vi "Virtual Oscilloscope.vi"() -> ()   [LabVIEW 2017]
uses:
  Control 3.ctl
  Virt.Scope.ctl
  <instrlib>/Tektronix TDS 200 1000 2000 Series/Public/Configure/Configure Trigger (Edge).vi
  <instrlib>/Tektronix TDS 200 1000 2000 Series/Tektronix TDS 200 1000 2000 Series.lvlib
panel:
  in  "Rising/Falling":u16(ring) items=["Rising", "Falling"]
  out "Waveform Graph 2":waveform(dbl)(graph)={"t0"=timestamp(-0.050000000000000044 s since 1904-01-01), "dt"=4e-05, "Y"=[]}
  out "Waveform Graph":waveform(dbl)(graph)
  in  "Meas. Type":T1
  out "Measurement":dbl=21.349275589
  in  "stop":bool
  in  "Measure":bool
  in  "Voltage Scale 2":dbl(ring)=5.0 items=["50 V"=50.0, "20 V"=20.0, "10 V"=10.0, "5 V"=5.0, "2 V"=2.0, "1 V"=1.0, "500 mV"=0.5, "200 mV"=0.2, "100 mV"=0.1, "50 mV"=0.05, "20 mV"=0.02]
  in  "Voltage Scale 1":dbl(ring)=10.0 items=["50 V"=50.0, "20 V"=20.0, "10 V"=10.0, "5 V"=5.0, "2 V"=2.0, "1 V"=1.0, "500 mV"=0.5, "200 mV"=0.2, "100 mV"=0.1, "50 mV"=0.05, "20 mV"=0.02]
  in  "Horz Trigger":dbl min=-1.0 max=1.0 step=0.001
  in  "Vert Trigger":dbl min=-200.0 max=200.0 step=1.0
  in  "Time Scale":dbl(ring)=0.01 items=["50 s"=50.0, "25 s"=25.0, "10 s"=10.0, "5 s"=5.0, "2.50 s"=2.5, "1 s"=1.0, "500 ms"=0.5, "250 ms"=0.25, "100 ms"=0.1, "50 ms"=0.05, "25 ms"=0.025, "10 ms"=0.01, "5 ms"=0.005, "2.50 ms"=0.0025, "1 ms"=0.001, "500 us"=0.0005, "250 us"=0.00025, "100 us"=0.0001, "50 us"=5e-05, "25 us"=2.5e-05, "10 us"=1e-05, "5 us"=5e-06, "2.50 us"=2.5e-06, "1 us"=1e-06, "500 ns"=5e-07, "250 ns"=2.5e-07, "100 ns"=1e-07, "50 ns"=5e-08, "25 ns"=2.5e-08, "10 ns"=1e-08, "5 ns"=5e-09]
  in  "Auto Set":bool
  # "Vertical"
  # "Horizontal"
  # "Ch 1"
  # "Ch 2"
  # "s"
  # "V"
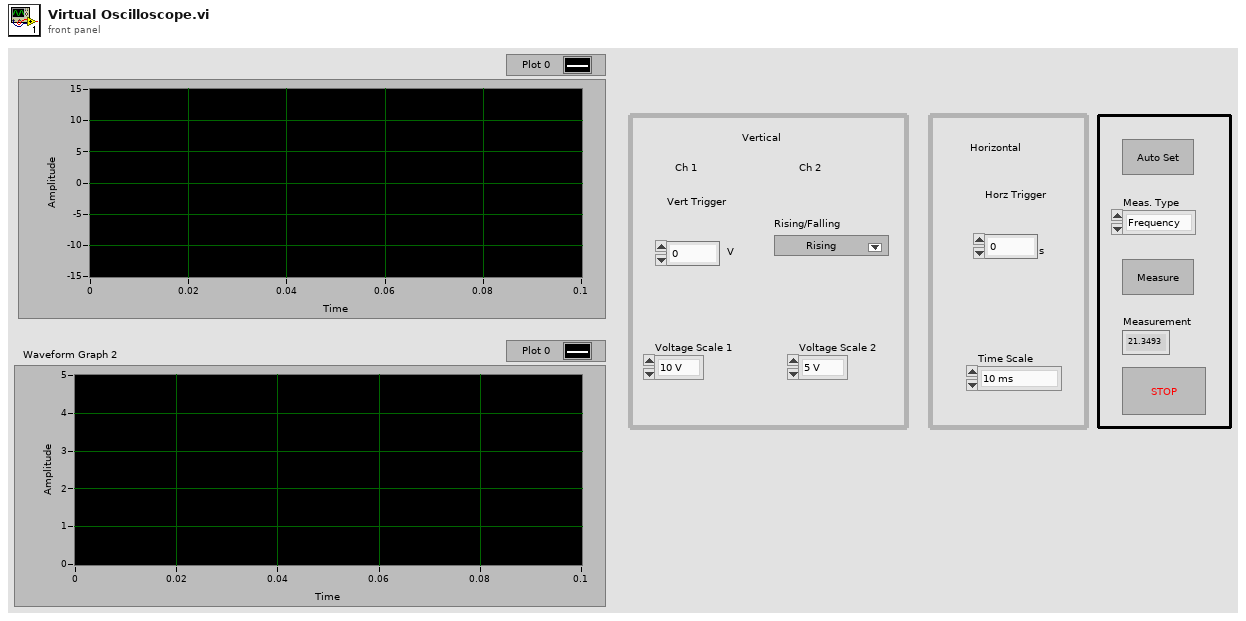
[diagram p1: front panel]
types:
  T1 = typedef "Control 3.ctl" = enum16{"Frequency", "Period", "PK-PK", "Cycle RMS"}
  T2 = typedef "Virt.Scope.ctl" = enum16{"Initialize", "Wait For UI", "Update", "Auto Set", "Read", "Display", "Stop"}
  T3 = cluster{"Baud Rate":u32, "Parity":u16, "Stop Bits":u16, "Flow Control":u16}
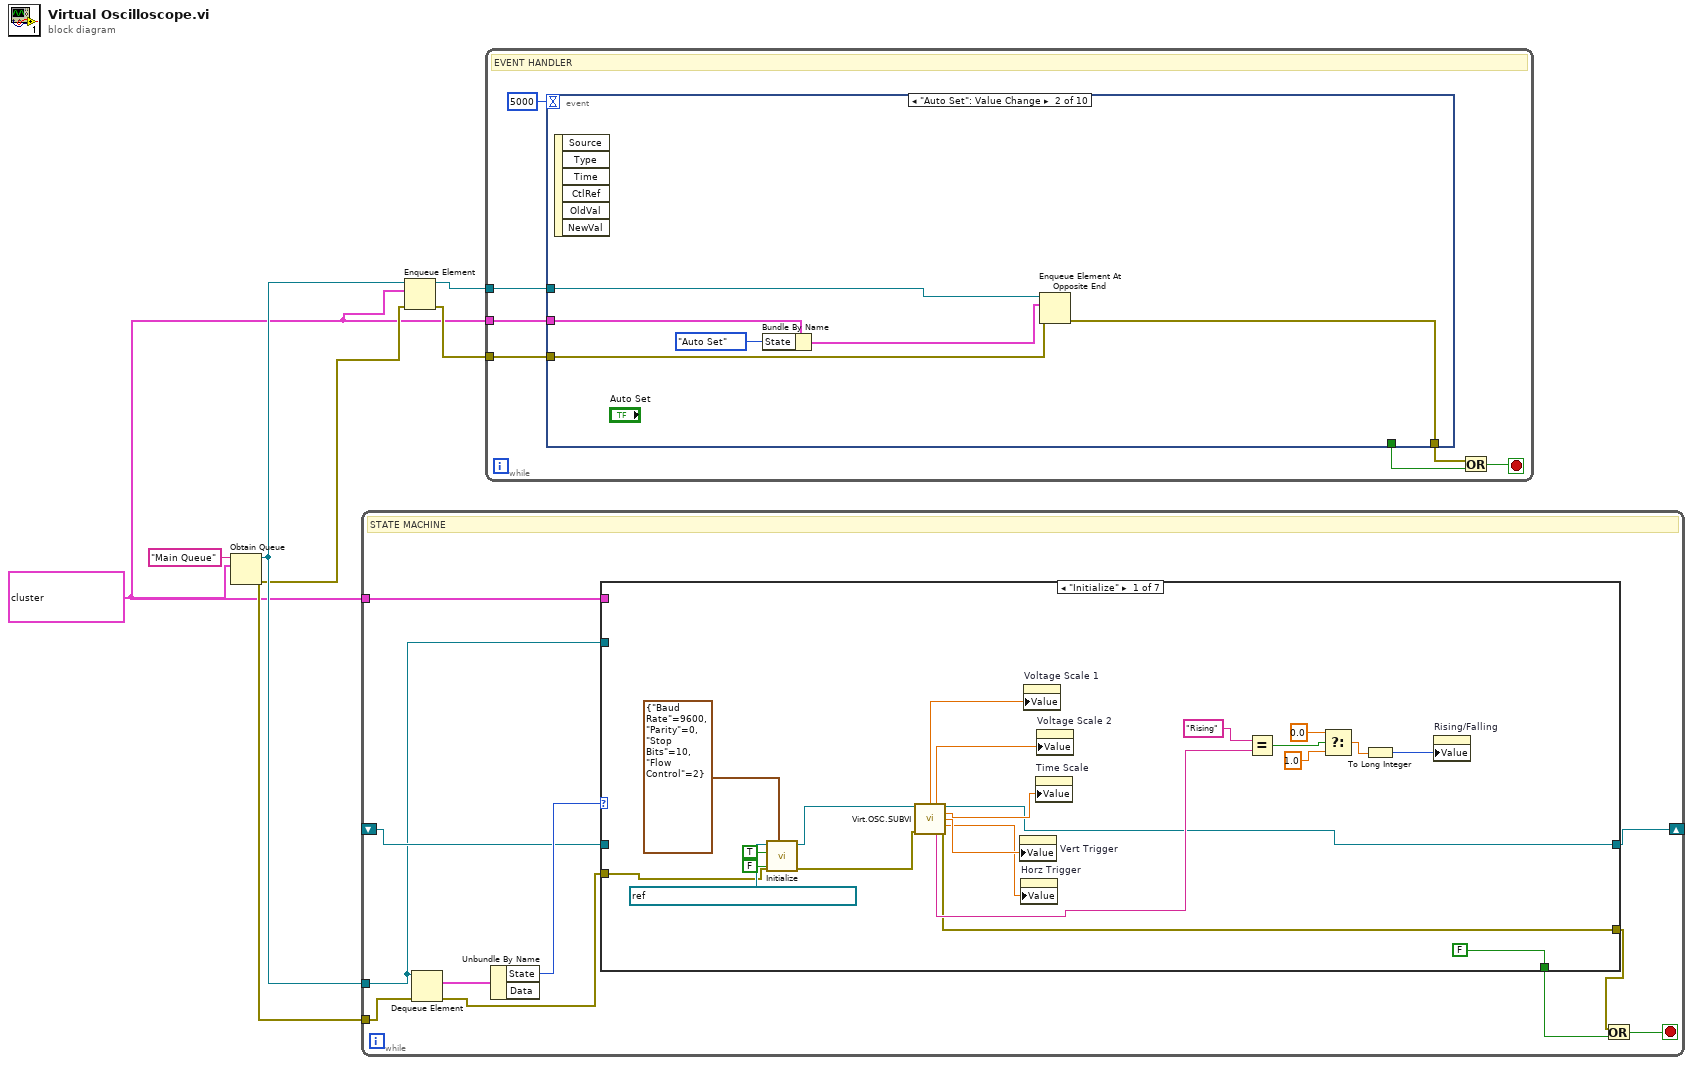
[diagram p0: block diagram]
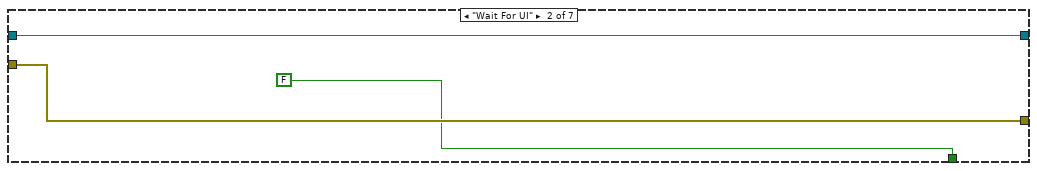
[diagram p2: hidden frame]
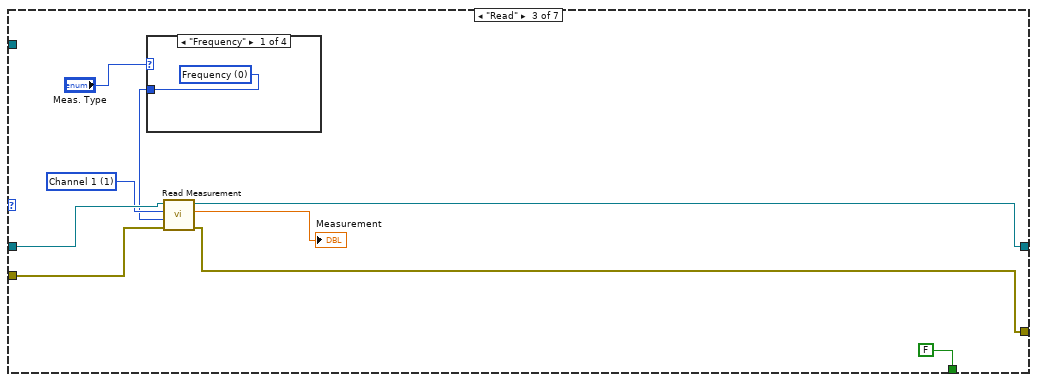
[diagram p3: hidden frame]
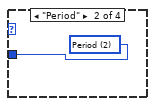
[diagram p4: hidden frame]
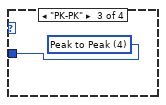
[diagram p5: hidden frame]
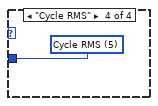
[diagram p6: hidden frame]
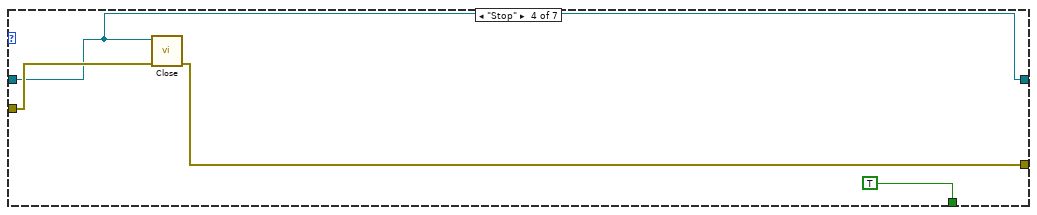
[diagram p7: hidden frame]
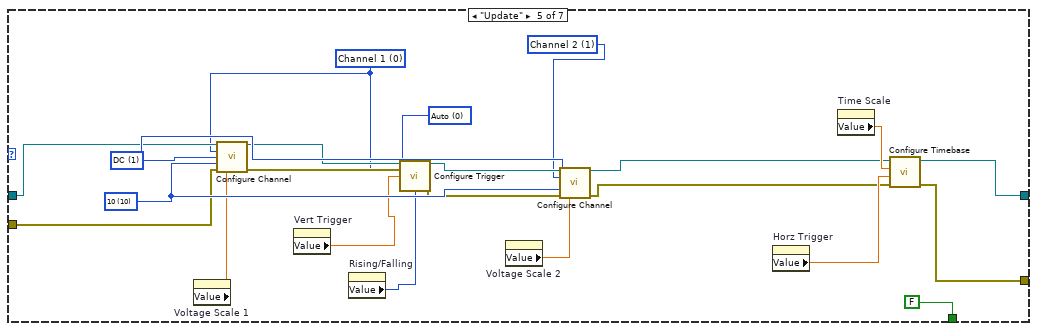
[diagram p8: hidden frame]
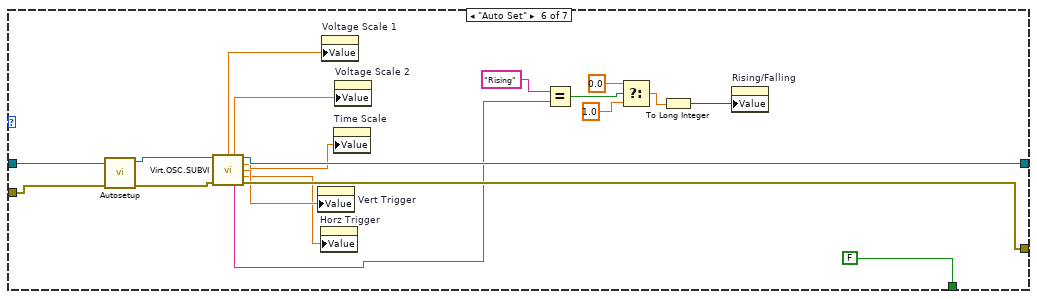
[diagram p9: hidden frame]
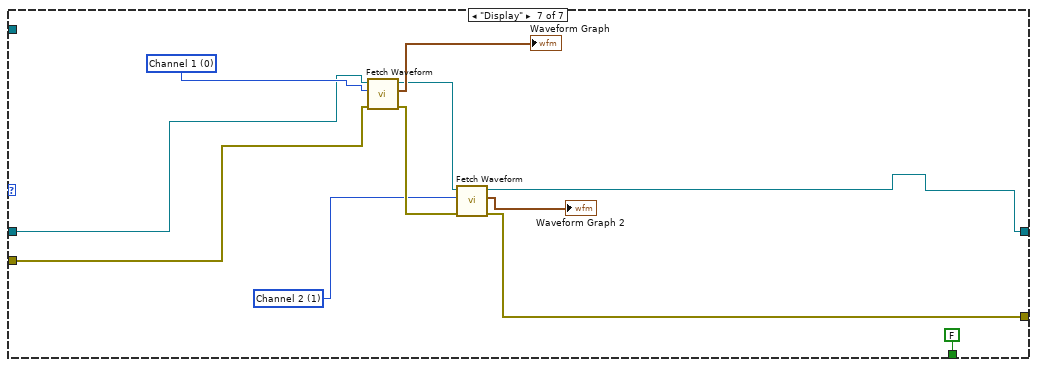
[diagram p10: hidden frame]
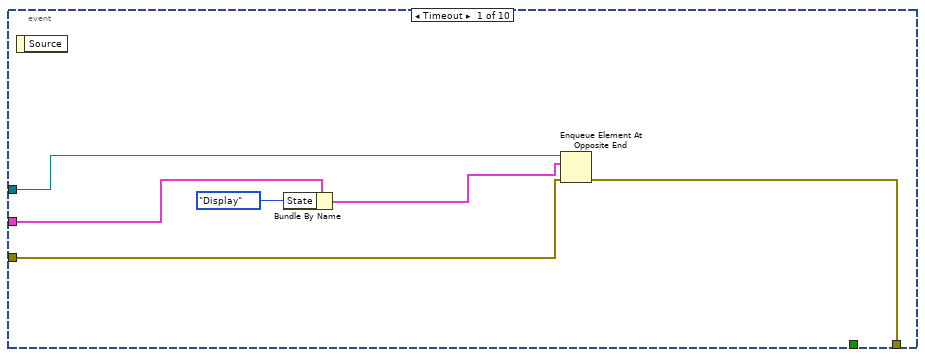
[diagram p11: hidden frame]
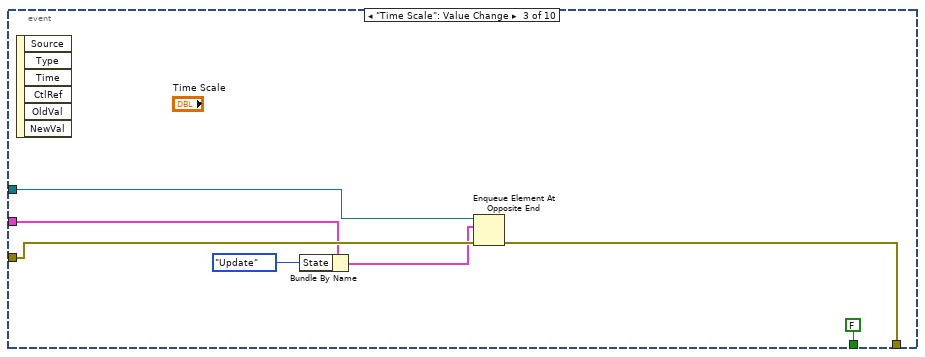
[diagram p12: hidden frame]
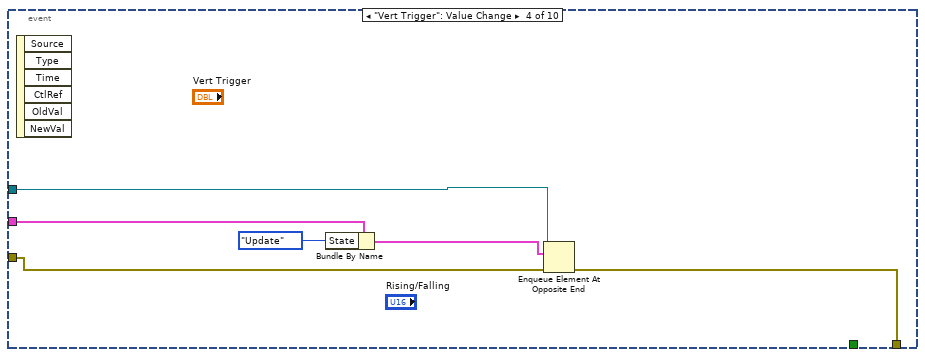
[diagram p13: hidden frame]
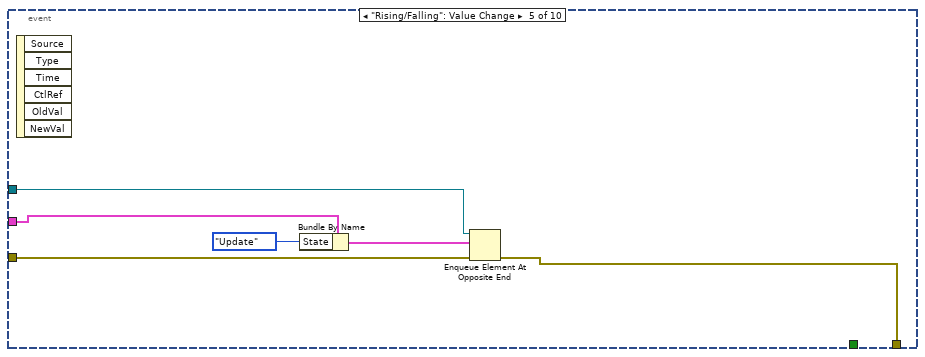
[diagram p14: hidden frame]
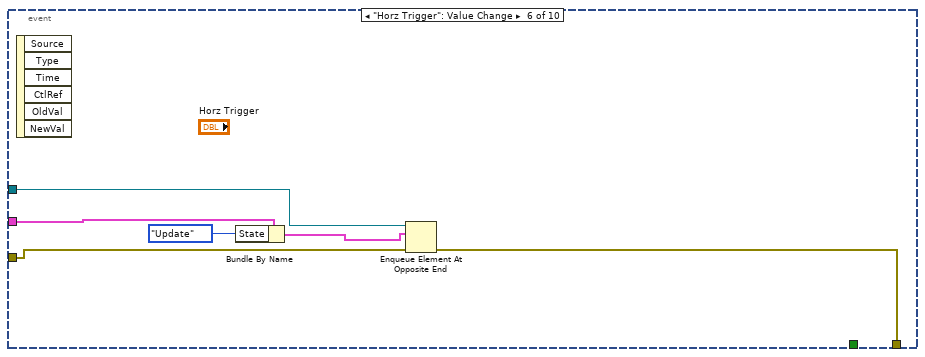
[diagram p15: hidden frame]
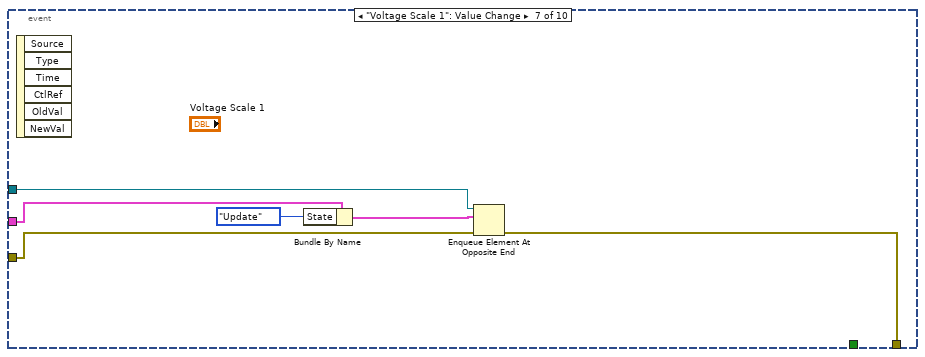
[diagram p16: hidden frame]
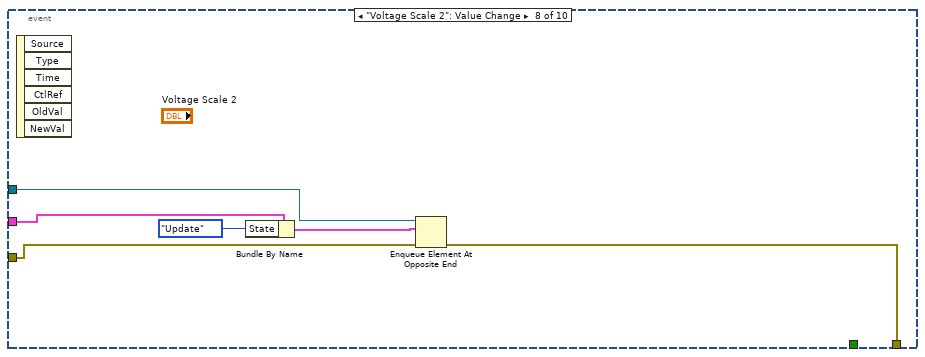
[diagram p17: hidden frame]
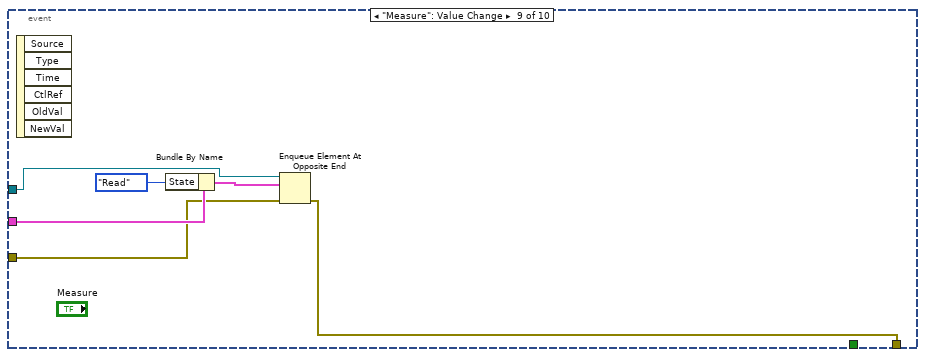
[diagram p18: hidden frame]
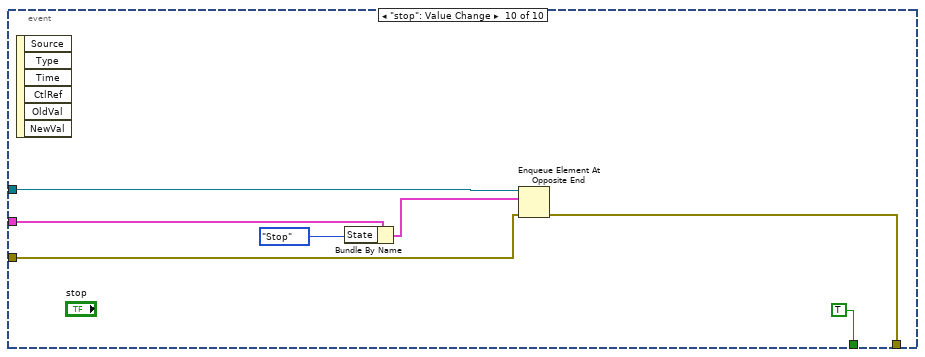
[diagram p19: hidden frame]
diagram:
  w1 = cluster{"Data":variant, "State":T2} {"Data"=variant, "State"=enum."Initialize"}
  n1 = Obtain Queue(name (unnamed)="Main Queue", element data type=w1) -> (queue out=w5:refnum<queue>, error out=w3:errorcluster)  [unwired: 3 in, 1 out]
  n2 = while {
    tunnel: w3 -> [w16]
    tunnel: w5 -> [w9]
    shift-right: [w7] -> _
    shift-left: _ -> [w11]
    tunnel: w1 -> [w8]
    stop <- w17 stop-if-true
    # "STATE MACHINE"
    n3 = Dequeue Element(queue=w9, error in (no error)=w16) -> (element=w15:cluster{"Data":variant, "State":T2}, error out=w13:errorcluster)  [unwired: 1 in, 2 out]
    n4 = Unbundle By Name(w15) -> ("State"=w14:T2)  [unwired: 1 out]
    n5 = case shown="\"Initialize\"" w14 {
      tunnel: w13 -> [w36 w41 w46 w59 w72 w98 w108]
      tunnel: [w19 w41 w44 w58 w71 w94 w102] -> w12
      tunnel: [w20 w42 w45 w56 w78 w95 w103] -> w7
      tunnel: w11 -> [_ w42 w51 w56 w73 w99 w109]
      tunnel: [FALSE FALSE FALSE TRUE FALSE FALSE FALSE] -> w10
      tunnel: w9 -> [_ _ _ _ _ _ _]
      tunnel: w8 -> [_ _ _ _ _ _ _]
      frame "Initialize" {
        n6 = call <instrlib>:"Initialize.vi"("Serial Configuration"=T3 {"Baud Rate"=9600, "Parity"=0, "Stop Bits"=10, "Flow Control"=2}, "error in (no error)"=w36, "Reset? (T: Yes)"=FALSE, "ID Query? (T: Yes)"=TRUE, "VISA resource name"=refnum<visa-resource-name> "USB0::0x0699::0x03A0::C014023::INSTR") -> ("error out"=w21:errorcluster, "VISA resource name out"=w22:refnum<visa-resource-name>)  [unwired: 5 in]
        n7 = call "Virt.OSC.SUBVI.vi"("VISA resource name"=w22, "Error In"=w21) -> ("Channel 1 Scale"=w33:dbl, "Channel 2 Scale"=w32:dbl, "VISA resource name out"=w20:refnum<visa-resource-name>, "Time Base"=w31:dbl, "vertical trigger"=w30:dbl, "horziontal trigger"=w18:dbl, "rise/fall"=w29:string, "Error Out"=w19:errorcluster)  [unwired: 6 in]
        n8 = property on="Vert Trigger" class="DigNum (strict)"("Value"=w30) -> ()  [unwired: 2 in, 2 out]
        n9 = property on="Horz Trigger" class="DigNum (strict)"("Value"=w18) -> ()  [unwired: 2 in, 2 out]
        n10 = property on="Voltage Scale 1" class="Ring (strict)"("Value"=w33) -> ()  [unwired: 2 in, 2 out]
        n11 = property on="Time Scale" class="Ring (strict)"("Value"=w31) -> ()  [unwired: 2 in, 2 out]
        n12 = property on="Voltage Scale 2" class="Ring (strict)"("Value"=w32) -> ()  [unwired: 2 in, 2 out]
        n13 = Equal?(x="Rising", y=w29) -> (x = y?=w28:bool)
        n14 = Select(t=0.0, s=w28, f=1.0) -> (s? t:f=w27:dbl)
        n15 = To Long Integer(number=w27) -> (32bit integer=w26:i32)
        n16 = property on="Rising/Falling" class="Ring (strict)"("Value"=w26) -> ()  [unwired: 2 in, 2 out]
      }
      frame "Wait For UI" {
      }
      frame "Read" {
        w50 = 1 items=["Channel 1"=1, "Channel 2"=2, "Channel 3"=3, "Channel 4"=4] ("Channel (1: Channel 1)")
        n17 = case shown="\"Frequency\"" "Meas. Type" {
          tunnel: [w52 w53 w54 w55] -> w47
          frame "Frequency" {
            w52 = 0 items=["Frequency", "Mean", "Period", "Pulse Duty", "Peak to Peak", "Cycle RMS", "Minimum", "Maximum", "Rise Time", "Fall Time", "Positive Width", "Negative Width", "Amplitude", "Cycle Mean", "High", "Low", "Negative Duty", "Positive Overshoot", "Negative Overshoot", "Cursor Mean", "Burst Width", "Positive Pulse Count", "Negative Pulse Count", "Rising Edge Count", "Falling Edge Count", "Area", "Cycle Area", "RMS", "Cursor RMS"] ("Measurement Type (0: Frequency)")
          }
          frame "Period" {
            w53 = 2 items=["Frequency", "Mean", "Period", "Pulse Duty", "Peak to Peak", "Cycle RMS", "Minimum", "Maximum", "Rise Time", "Fall Time", "Positive Width", "Negative Width", "Amplitude", "Cycle Mean", "High", "Low", "Negative Duty", "Positive Overshoot", "Negative Overshoot", "Cursor Mean", "Burst Width", "Positive Pulse Count", "Negative Pulse Count", "Rising Edge Count", "Falling Edge Count", "Area", "Cycle Area", "RMS", "Cursor RMS"] ("Measurement Type (0: Frequency)")
          }
          frame "PK-PK" {
            w54 = 4 items=["Frequency", "Mean", "Period", "Pulse Duty", "Peak to Peak", "Cycle RMS", "Minimum", "Maximum", "Rise Time", "Fall Time", "Positive Width", "Negative Width", "Amplitude", "Cycle Mean", "High", "Low", "Negative Duty", "Positive Overshoot", "Negative Overshoot", "Cursor Mean", "Burst Width", "Positive Pulse Count", "Negative Pulse Count", "Rising Edge Count", "Falling Edge Count", "Area", "Cycle Area", "RMS", "Cursor RMS"] ("Measurement Type (0: Frequency)")
          }
          frame "Cycle RMS" {
            w55 = 5 items=["Frequency", "Mean", "Period", "Pulse Duty", "Peak to Peak", "Cycle RMS", "Minimum", "Maximum", "Rise Time", "Fall Time", "Positive Width", "Negative Width", "Amplitude", "Cycle Mean", "High", "Low", "Negative Duty", "Positive Overshoot", "Negative Overshoot", "Cursor Mean", "Burst Width", "Positive Pulse Count", "Negative Pulse Count", "Rising Edge Count", "Falling Edge Count", "Area", "Cycle Area", "RMS", "Cursor RMS"] ("Measurement Type (0: Frequency)")
          }
        }
        n18 = call <instrlib>:"Read Measurement.vi"("error in (no error)"=w46, "Measurement Type (0: Frequency)"=w47, "Channel (1: Channel 1)"=w50, "VISA resource name"=w51) -> ("error out"=w44:errorcluster, "Measurement"=→"Measurement":dbl, "VISA resource name out"=w45:refnum<visa-resource-name>)  [unwired: 4 in, 1 out]
      }
      frame "Stop" {
        n19 = call <instrlib>:"Close.vi"("error in (no error)"=w59, "VISA resource name"=w56) -> ("error out"=w58:errorcluster)  [unwired: 9 in]
      }
      frame "Update" {
        w63 = 0 items=["Auto", "Normal"] ("Trigger Mode (0: Auto)")
        w64 = 1 items=["Channel 1", "Channel 2", "Channel 3", "Channel 4", "Math", "Reference A", "Reference B", "Reference C", "Reference D"] ("Channel (0: Channel 1)")
        w79 = 10 items=["1"=1, "10"=10, "20"=20, "50"=50, "100"=100, "500"=500, "1000"=1000] ("Probe Attenuation (10: 10X)")
        w80 = 1 items=["AC", "DC", "Ground"] ("Vertical Coupling (1: DC)")
        w66 = 0 items=["Channel 1", "Channel 2", "Channel 3", "Channel 4", "Math", "Reference A", "Reference B", "Reference C", "Reference D"] ("Channel (0: Channel 1)")
        n20 = property on="Voltage Scale 1" class="Ring (strict)"() -> ("Value"=w77:dbl)  [unwired: 2 in, 2 out]
        n21 = call <instrlib>:"Configure Channel.vi"("VISA resource name"=w73, "Channel (0: Channel 1)"=w66, "Vertical Coupling (1: DC)"=w80, "Probe Attenuation (10: 10X)"=w79, "error in (no error)"=w72, "Vertical Range (10.0 V/div)"=w77) -> ("VISA resource name out"=w70:refnum<visa-resource-name>, "error out"=w69:errorcluster)  [unwired: 8 in]
        n22 = property on="Vert Trigger" class="DigNum (strict)"() -> ("Value"=w65:dbl)  [unwired: 2 in, 2 out]
        n23 = property on="Rising/Falling" class="Ring (strict)"() -> ("Value"=w62:u16)  [unwired: 2 in, 2 out]
        n24 = call-poly <instrlib>:"Configure Trigger.vi"("VISA resource name"=w70, "Trigger Source (0: Channel 1)"=w66, "Trigger Level (0.0 V)"=w65, "Trigger Mode (0: Auto)"=w63, "error in (no error)"=w69, "Trigger Slope (0: Rising)"=w62) -> ("VISA resource name out"=w67:refnum<visa-resource-name>, "error out"=w68:errorcluster)  [unwired: 8 in]
        n25 = property on="Voltage Scale 2" class="Ring (strict)"() -> ("Value"=w76:dbl)  [unwired: 2 in, 2 out]
        n26 = call <instrlib>:"Configure Channel.vi"("VISA resource name"=w67, "Channel (0: Channel 1)"=w64, "Vertical Coupling (1: DC)"=w80, "Probe Attenuation (10: 10X)"=w79, "error in (no error)"=w68, "Vertical Range (10.0 V/div)"=w76) -> ("VISA resource name out"=w61:refnum<visa-resource-name>, "error out"=w60:errorcluster)  [unwired: 8 in]
        n27 = property on="Horz Trigger" class="DigNum (strict)"() -> ("Value"=w75:dbl)  [unwired: 2 in, 2 out]
        n28 = property on="Time Scale" class="Ring (strict)"() -> ("Value"=w74:dbl)  [unwired: 2 in, 2 out]
        n29 = call <instrlib>:"Configure Timebase.vi"("error in (no error)"=w60, "Position (0.0 s)"=w75, "Timebase (0.0005 s)"=w74, "VISA resource name"=w61) -> ("error out"=w71:errorcluster, "VISA resource name out"=w78:refnum<visa-resource-name>)  [unwired: 6 in]
      }
      frame "Auto Set" {
        n30 = call <instrlib>:"Autosetup.vi"("error in (no error)"=w98, "VISA resource name"=w99) -> ("error out"=w96:errorcluster, "VISA resource name out"=w97:refnum<visa-resource-name>)  [unwired: 8 in]
        n31 = call "Virt.OSC.SUBVI.vi"("VISA resource name"=w97, "Error In"=w96) -> ("Channel 1 Scale"=w93:dbl, "Channel 2 Scale"=w92:dbl, "VISA resource name out"=w95:refnum<visa-resource-name>, "Time Base"=w91:dbl, "vertical trigger"=w90:dbl, "horziontal trigger"=w82:dbl, "rise/fall"=w89:string, "Error Out"=w94:errorcluster)  [unwired: 6 in]
        n32 = property on="Vert Trigger" class="DigNum (strict)"("Value"=w90) -> ()  [unwired: 2 in, 2 out]
        n33 = property on="Horz Trigger" class="DigNum (strict)"("Value"=w82) -> ()  [unwired: 2 in, 2 out]
        n34 = property on="Voltage Scale 1" class="Ring (strict)"("Value"=w93) -> ()  [unwired: 2 in, 2 out]
        n35 = property on="Time Scale" class="Ring (strict)"("Value"=w91) -> ()  [unwired: 2 in, 2 out]
        n36 = property on="Voltage Scale 2" class="Ring (strict)"("Value"=w92) -> ()  [unwired: 2 in, 2 out]
        n37 = Equal?(x="Rising", y=w89) -> (x = y?=w87:bool)
        n38 = Select(t=0.0, s=w87, f=1.0) -> (s? t:f=w86:dbl)
        n39 = To Long Integer(number=w86) -> (32bit integer=w83:i32)
        n40 = property on="Rising/Falling" class="Ring (strict)"("Value"=w83) -> ()  [unwired: 2 in, 2 out]
      }
      frame "Display" {
        w104 = u16 1 items=["Channel 1", "Channel 2", "Channel 3", "Channel 4", "Math", "Reference A", "Reference B", "Reference C", "Reference D", "FFT"] ("Source (0: Channel 1)")
        w110 = u16 0 items=["Channel 1", "Channel 2", "Channel 3", "Channel 4", "Math", "Reference A", "Reference B", "Reference C", "Reference D", "FFT"] ("Source (0: Channel 1)")
        n41 = call <instrlib>:"Fetch Waveform.vi"("error in (no error)"=w108, "Source (0: Channel 1)"=w110, "VISA resource name"=w109) -> ("error out"=w106:errorcluster, "Waveform Data"=→"Waveform Graph":waveform(dbl), "VISA resource name out"=w105:refnum<visa-resource-name>)  [unwired: 6 in]
        n42 = call <instrlib>:"Fetch Waveform.vi"("error in (no error)"=w106, "Source (0: Channel 1)"=w104, "VISA resource name"=w105) -> ("error out"=w102:errorcluster, "Waveform Data"=→"Waveform Graph 2":waveform(dbl), "VISA resource name out"=w103:refnum<visa-resource-name>)  [unwired: 6 in]
      }
    }
    n43 = Or(x=w12, y=w10) -> (x .or. y?=w17:bool)
  }
  n44 = Enqueue Element(queue=w5, element=w1, error in (no error)=w3) -> (queue out=w4:refnum<queue>, error out=w2:errorcluster)  [unwired: 1 in, 1 out]
  n45 = while {
    tunnel: w2 -> [w116]
    tunnel: w4 -> [w117]
    tunnel: w1 -> [w118]
    stop <- w115 stop-if-true
    # "EVENT HANDLER"
    n46 = event shown="[1] \"Auto Set\": Value Change" {
      selector: _ -> [_ _ _ _ _ _ _ _ _ _]
      dyn-events: _ -> [_ _ _ _ _ _ _ _ _ _]
      timeout: 5000 -> [_ _ _ _ _ _ _ _ _ _]
      tunnel: w118 -> [w122 w128 w135 w141 w147 w152 w158 w165 w172 w177]
      tunnel: w117 -> [w123 w129 w133 w140 w148 w153 w159 w164 w173 w180]
      tunnel: w116 -> [w121 w127 w136 w142 w145 w151 w157 w163 w171 w179]
      tunnel: [_ _ FALSE _ _ _ _ _ _ TRUE] -> w114
      tunnel: [w119 w125 w132 w138 w144 w150 w156 w162 w168 w174] -> w113
      event Timeout {
        n47 = event-data() -> ()  [unwired: 1 in, 1 out]
        n48 = Bundle By Name(cluster=w122, "State"=Virt.Scope."Display") -> (w120:cluster{"Data":variant, "State":T2})
        n49 = Enqueue Element At Opposite End(queue=w123, element=w120, error in (no error)=w121) -> (error out=w119:errorcluster)  [unwired: 1 in, 2 out]
      }
      event "Auto Set": Value Change {
        n50 = event-data() -> ()  [unwired: 1 in, 6 out]
        n51 = Bundle By Name(cluster=w128, "State"=Virt.Scope."Auto Set") -> (w126:cluster{"Data":variant, "State":T2})
        n52 = Enqueue Element At Opposite End(queue=w129, element=w126, error in (no error)=w127) -> (error out=w125:errorcluster)  [unwired: 1 in, 2 out]
      }
      event "Time Scale": Value Change {
        n53 = event-data() -> ()  [unwired: 1 in, 6 out]
        n54 = Bundle By Name(cluster=w135, "State"=Virt.Scope."Update") -> (w134:cluster{"Data":variant, "State":T2})
        n55 = Enqueue Element At Opposite End(queue=w133, element=w134, error in (no error)=w136) -> (error out=w132:errorcluster)  [unwired: 1 in, 2 out]
      }
      event "Vert Trigger": Value Change {
        n56 = event-data() -> ()  [unwired: 1 in, 6 out]
        n57 = Bundle By Name(cluster=w141, "State"=Virt.Scope."Update") -> (w139:cluster{"Data":variant, "State":T2})
        n58 = Enqueue Element At Opposite End(queue=w140, element=w139, error in (no error)=w142) -> (error out=w138:errorcluster)  [unwired: 1 in, 2 out]
      }
      event "Rising/Falling": Value Change {
        n59 = event-data() -> ()  [unwired: 1 in, 6 out]
        n60 = Bundle By Name(cluster=w147, "State"=Virt.Scope."Update") -> (w146:cluster{"Data":variant, "State":T2})
        n61 = Enqueue Element At Opposite End(queue=w148, element=w146, error in (no error)=w145) -> (error out=w144:errorcluster)  [unwired: 1 in, 2 out]
      }
      event "Horz Trigger": Value Change {
        n62 = event-data() -> ()  [unwired: 1 in, 6 out]
        n63 = Bundle By Name(cluster=w152, "State"=Virt.Scope."Update") -> (w154:cluster{"Data":variant, "State":T2})
        n64 = Enqueue Element At Opposite End(queue=w153, element=w154, error in (no error)=w151) -> (error out=w150:errorcluster)  [unwired: 1 in, 2 out]
      }
      event "Voltage Scale 1": Value Change {
        n65 = event-data() -> ()  [unwired: 1 in, 6 out]
        n66 = Bundle By Name(cluster=w158, "State"=Virt.Scope."Update") -> (w160:cluster{"Data":variant, "State":T2})
        n67 = Enqueue Element At Opposite End(queue=w159, element=w160, error in (no error)=w157) -> (error out=w156:errorcluster)  [unwired: 1 in, 2 out]
      }
      event "Voltage Scale 2": Value Change {
        n68 = event-data() -> ()  [unwired: 1 in, 6 out]
        n69 = Bundle By Name(cluster=w165, "State"=Virt.Scope."Update") -> (w166:cluster{"Data":variant, "State":T2})
        n70 = Enqueue Element At Opposite End(queue=w164, element=w166, error in (no error)=w163) -> (error out=w162:errorcluster)  [unwired: 1 in, 2 out]
      }
      event "Measure": Value Change {
        n71 = event-data() -> ()  [unwired: 1 in, 6 out]
        n72 = Bundle By Name(cluster=w172, "State"=Virt.Scope."Read") -> (w170:cluster{"Data":variant, "State":T2})
        n73 = Enqueue Element At Opposite End(queue=w173, element=w170, error in (no error)=w171) -> (error out=w168:errorcluster)  [unwired: 1 in, 2 out]
      }
      event "stop": Value Change {
        n74 = event-data() -> ()  [unwired: 1 in, 6 out]
        n75 = Bundle By Name(cluster=w177, "State"=Virt.Scope."Stop") -> (w176:cluster{"Data":variant, "State":T2})
        n76 = Enqueue Element At Opposite End(queue=w180, element=w176, error in (no error)=w179) -> (error out=w174:errorcluster)  [unwired: 1 in, 2 out]
      }
    }
    n77 = Or(x=w113, y=w114) -> (x .or. y?=w115:bool)
  }
